vi "Resolve-client-from-identifier.vi"(8 "error in (no error)":errorcluster, 10 "Client identifier":string) -> (0 "error out":errorcluster, 1 "Client ID":i32, 2 "Client type":T1)   [LabVIEW 2013, in "PowderDeposition.lvlib" / "PD-Client.lvclass"]
uses:
  PD-Client.lvclass
  Supported-modules.ctl
  Custom-errors.ctl
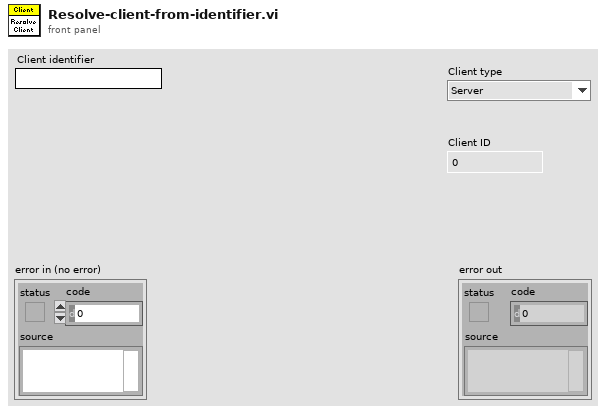
[diagram p1: front panel]
types:
  T1 = typedef "PowderDeposition.lvlib/PD-Client.lvclass/Supported-modules.ctl" = enum16{"Server", "All", "SLMControl", "PowderDeposition", "StrategyParser", "CameraVision", "MaterialCharacterization", "StatusMonitor", "SLMSimulation", "LaserCharacterization"}
  T2 = typedef "PowderDeposition.lvlib/PD-Client.lvclass/Custom-errors.ctl" = enum16{"No error", "Command not recognized", "Invalid input", "Timeout", "Not implemented", "Unsupported message", "Unsupported client", "Unsupported action"}
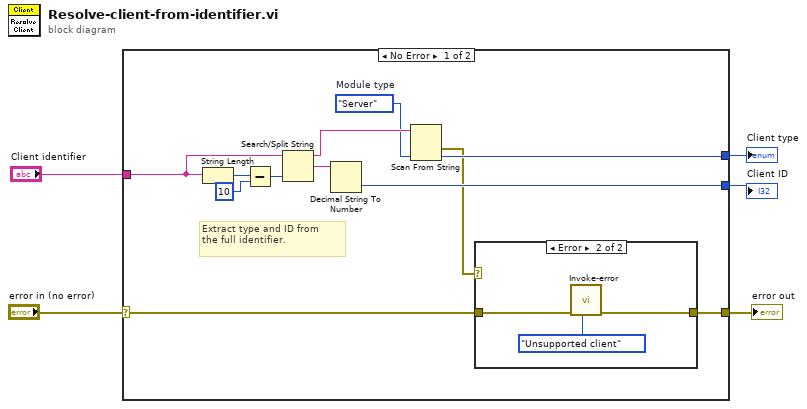
[diagram p0: block diagram]
diagram:
  n1 = case shown="No Error" "error in (no error)" {
    selector: "error in (no error)" -> [w7 w22]
    tunnel: [w6 w22] -> w4
    tunnel: "Client identifier" -> [w12 _]
    tunnel: [w9 _] -> w2
    tunnel: [w13 _] -> w1
    frame No Error {
      w10 = Supported-modules."Server"  # Module type
      # "Extract type and ID from\nthe full identifier."
      n2 = String Length(string=w12) -> (length=w17:i32)
      n3 = Subtract(x=w17, y=10) -> (x-y=w15:i32)
      n4 = Search/Split String(string=w12, offset (0)=w15) -> (substring before match=w11:string, match + rest of string=w14:string)  [unwired: 1 in, 1 out]
      n5 = Decimal String To Number(string=w14) -> (number=w13:i32)  [unwired: 2 in, 1 out]
      n6 = Scan From String(input string=w11, default 1=w10) -> (error out=w8:errorcluster, output 1=w9:T1)  [unwired: 3 in, 2 out]
      n7 = case shown="Error" w8 {
        tunnel: w7 -> [w18 w21]
        tunnel: [w18 w20] -> w6
        frame No Error {
        }
        frame Error {
          n8 = call "Invoke-error.vi"("Error"=Custom-errors."Unsupported client", "error in (no error)"=w21) -> ("error out"=w20:errorcluster)  [unwired: 9 in]
        }
      }
    }
    frame Error {
    }
  }
  "error out" <- w4
  "Client type" <- w2
  "Client ID" <- w1
